vi "Stack Control - Servo Flipper.vi"() -> ()   [LabVIEW 2012]
uses:
  BotStatus.vi
  Motors Values.vi
panel:
  in  "Suck":bool
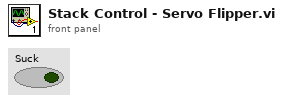
[diagram p1: front panel]
types:
  T1 = cluster{"Middle":bool, "InCannon":bool, "InFlipper":bool, "FlipperAtPlace":bool, "Bottom":bool, "FrisbeeDirection":bool}
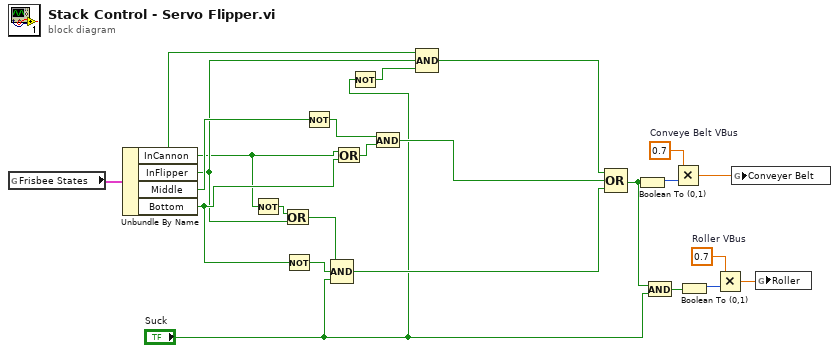
[diagram p0: block diagram]
diagram:
  w6 = 0.7  # Roller VBus
  w8 = 0.7  # Conveye Belt VBus
  n1 = global read "BotStatus.vi" "Frisbee States"() -> (w23:T1)
  n2 = Unbundle By Name(w23) -> ("InCannon"=w11:bool, "InFlipper"=w12:bool, "Middle"=w19:bool, "Bottom"=w16:bool)
  n3 = Not(x=w11) -> (.not. x?=w21:bool)
  n4 = Or(x=w21, y=w12) -> (x .or. y?=w20:bool)
  n5 = Not(x=w16) -> (.not. x?=w22:bool)
  n6 = Not(x=w19) -> (.not. x?=w18:bool)
  n7 = Compound Arithmetic op=AND(w20, w22, "Suck") -> (w14:bool)
  n8 = Or(x=w11, y=w16) -> (x .or. y?=w17:bool)
  n9 = Not(x="Suck") -> (.not. x?=w13:bool)
  n10 = And(x=w18, y=w17) -> (x .and. y?=w15:bool)
  n11 = Compound Arithmetic op=AND(w11, w12, w13) -> (w10:bool)
  n12 = Compound Arithmetic op=OR(w10, w15, w14) -> (w2:bool)
  n13 = Boolean To (0,1)(Boolean=w2) -> (0, 1=w9:i16)
  n14 = And(x=w2, y="Suck") -> (x .and. y?=w3:bool)
  n15 = Multiply(x=w8, y=w9) -> (x*y=w7:dbl)
  n16 = Boolean To (0,1)(Boolean=w3) -> (0, 1=w5:i16)
  n17 = Multiply(x=w6, y=w5) -> (x*y=w4:dbl)
  n18 = global write "Motors Values.vi" "Conveyer Belt"(w7) -> ()
  n19 = global write "Motors Values.vi" "Roller"(w4) -> ()
